vi "Benchmark Delete.vi"() -> ()   [LabVIEW 2017]
uses:
  Source/LookupTable/LookupTable.lvclass/LookupTable.ctl
  3f600695-5b5a-4146-a4af-1e267d96d976.vi
  b6b64ea5-f314-4d4f-8fa7-59ac42c8a07d.vi
  Source/LookupTable/Read Table Reference.vi
  Source/LookupTable/LookupTable.lvclass
panel:
  in  "Table Size":i32=100000
  out "Variant DVR":dbl
  out "Waveform Chart":cluster{dbl, dbl, dbl}(graph)
  out "Variant by value":dbl
  out "Composed Lookup Table":dbl
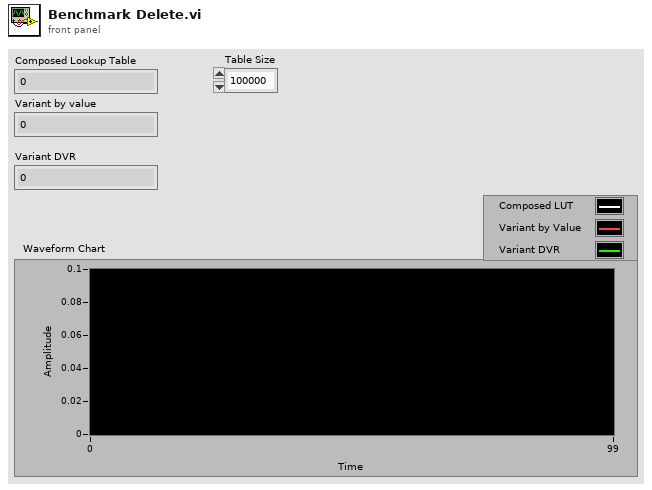
[diagram p1: front panel]
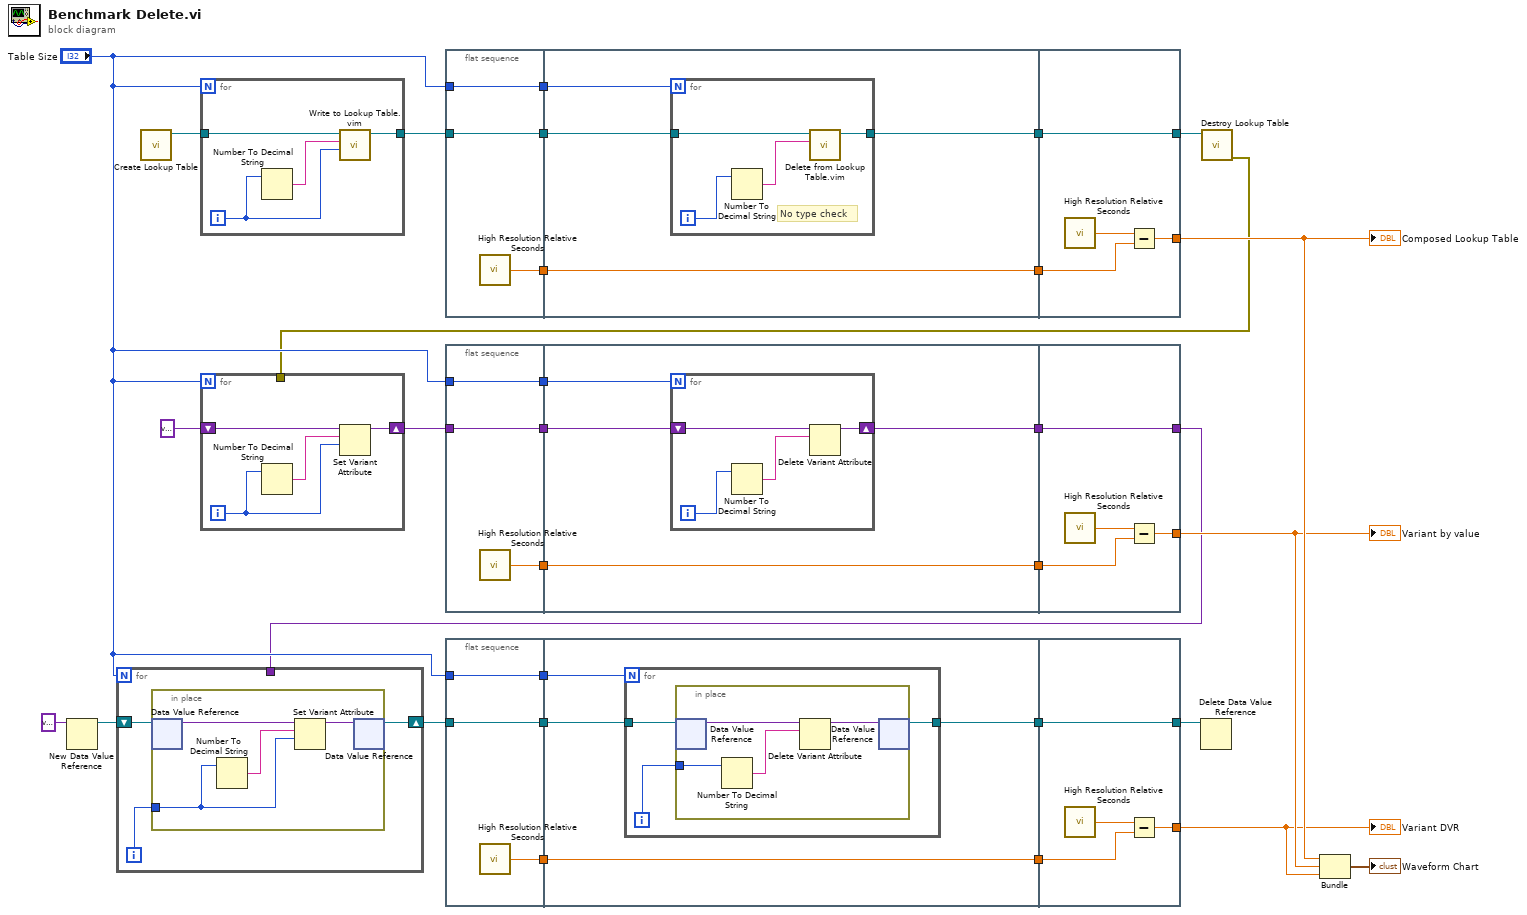
[diagram p0: block diagram]
diagram:
  n1 = New Data Value Reference(data value=variant) -> (data value reference=w12:refnum<data-value>)  [unwired: 1 in, 1 out]
  n2 = for {
    N: "Table Size" -> [_]
    shift-right: [w33] -> w11
    shift-left: w12 -> [w34]
    tunnel: w1 -> [_]
    i -> [w32]
    n3 = in-place {
      in-place-border: w32 -> [w35]
      n4 = in-place-dvr #1(w34) -> (w37:variant)  [unwired: 1 out]
      n5 = Number To Decimal String(number=w35) -> (decimal integer string=w38:string)  [unwired: 1 in]
      n6 = Set Variant Attribute(Variant=w37, name=w38, value=w35) -> (Variant out=w36:variant)  [unwired: 1 in, 2 out]
      n7 = in-place-dvr #1(w36) -> (w33:refnum<data-value>)  [unwired: 1 out]
    }
  }
  n8 = call "Create Lookup Table.vi"() -> ("LookupTable Reference"=w26:refnum<data-value>)  [unwired: 10 in, 1 out]
  n9 = for {
    N: "Table Size" -> [_]
    tunnel: [w40] -> w24
    tunnel: w26 -> [w39]
    i -> [w41]
    n10 = Number To Decimal String(number=w41) -> (decimal integer string=w42:string)  [unwired: 1 in]
    n11 = call "Write to Lookup Table.vim"("Item"=w41, "Item Name"=w42, "LookupTable Reference"=w39) -> ("LookupTable Reference Out"=w40:refnum<data-value>)  [unwired: 6 in, 2 out]
  }
  n12 = flat-sequence {
    tunnel: [w45] -> w31
    tunnel: [w44] -> w25
    tunnel: w24 -> [w44]
    tunnel: [w43] -> w19
    tunnel: "Table Size" -> [w43]
    tunnel: w31 -> [w49]
    tunnel: [w49] -> w30
    tunnel: w25 -> [w48]
    tunnel: [w47] -> w22
    tunnel: w19 -> [w46]
    tunnel: w30 -> [w56]
    tunnel: [w55] -> w9
    tunnel: [w54] -> w23
    tunnel: w22 -> [w54]
    frame #0 {
      n13 = call <vilib>:"High Resolution Relative Seconds.vi"() -> ("relative seconds"=w45:dbl)
    }
    frame #1 {
      n14 = for {
        N: w46 -> [_]
        tunnel: [w51] -> w47
        tunnel: w48 -> [w50]
        i -> [w52]
        # "No type check"
        n15 = Number To Decimal String(number=w52) -> (decimal integer string=w53:string)  [unwired: 1 in]
        n16 = call "Delete from Lookup Table.vim"("Item Name"=w53, "LookupTable Reference"=w50) -> ("LookupTable Reference Out"=w51:refnum<data-value>)  [unwired: 7 in, 2 out]
      }
    }
    frame #2 {
      n17 = call <vilib>:"High Resolution Relative Seconds.vi"() -> ("relative seconds"=w57:dbl)
      n18 = Subtract(x=w57, y=w56) -> (x-y=w55:dbl)
    }
  }
  n19 = flat-sequence {
    tunnel: [w60] -> w29
    tunnel: [w59] -> w21
    tunnel: w20 -> [w59]
    tunnel: "Table Size" -> [w58]
    tunnel: [w58] -> w18
    tunnel: w29 -> [w64]
    tunnel: [w64] -> w28
    tunnel: w21 -> [w63]
    tunnel: w18 -> [w62]
    tunnel: [w61] -> w3
    tunnel: w28 -> [w71]
    tunnel: [w70] -> w8
    tunnel: [w69] -> w1
    tunnel: w3 -> [w69]
    frame #0 {
      n20 = call <vilib>:"High Resolution Relative Seconds.vi"() -> ("relative seconds"=w60:dbl)
    }
    frame #1 {
      n21 = for {
        N: w62 -> [_]
        shift-right: [w68] -> w61
        shift-left: w63 -> [w65]
        i -> [w66]
        n22 = Number To Decimal String(number=w66) -> (decimal integer string=w67:string)  [unwired: 1 in]
        n23 = Delete Variant Attribute(6:w67, 7:w65) -> (3:w68:variant)  [unwired: 1 in, 2 out]
      }
    }
    frame #2 {
      n24 = call <vilib>:"High Resolution Relative Seconds.vi"() -> ("relative seconds"=w72:dbl)
      n25 = Subtract(x=w72, y=w71) -> (x-y=w70:dbl)
    }
  }
  n26 = flat-sequence {
    tunnel: [w75] -> w17
    tunnel: [w74] -> w16
    tunnel: w11 -> [w74]
    tunnel: "Table Size" -> [w73]
    tunnel: [w73] -> w15
    tunnel: w17 -> [w79]
    tunnel: [w79] -> w14
    tunnel: w16 -> [w78]
    tunnel: w15 -> [w76]
    tunnel: [w77] -> w4
    tunnel: w14 -> [w89]
    tunnel: [w88] -> w7
    tunnel: [w87] -> w5
    tunnel: w4 -> [w87]
    frame #0 {
      n27 = call <vilib>:"High Resolution Relative Seconds.vi"() -> ("relative seconds"=w75:dbl)
    }
    frame #1 {
      n28 = for {
        N: w76 -> [_]
        tunnel: [w81] -> w77
        tunnel: w78 -> [w80]
        i -> [w82]
        n29 = in-place {
          in-place-border: w82 -> [w85]
          n30 = in-place-dvr #2(w80) -> (w84:variant)  [unwired: 1 out]
          n31 = Number To Decimal String(number=w85) -> (decimal integer string=w86:string)  [unwired: 1 in]
          n32 = Delete Variant Attribute(6:w86, 7:w84) -> (3:w83:variant)  [unwired: 1 in, 2 out]
          n33 = in-place-dvr #2(w83) -> (w81:refnum<data-value>)  [unwired: 1 out]
        }
      }
    }
    frame #2 {
      n34 = call <vilib>:"High Resolution Relative Seconds.vi"() -> ("relative seconds"=w90:dbl)
      n35 = Subtract(x=w90, y=w89) -> (x-y=w88:dbl)
    }
  }
  n36 = Delete Data Value Reference(data value reference=w5) -> ()  [unwired: 1 in, 2 out]
  n37 = call "Destroy Lookup Table.vi"("LookupTable Reference"=w23) -> ("error out"=w2:errorcluster)  [unwired: 10 in]
  n38 = for {
    N: "Table Size" -> [_]
    shift-right: [w94] -> w20
    shift-left: variant -> [w91]
    tunnel: w2 -> [_]
    i -> [w92]
    n39 = Number To Decimal String(number=w92) -> (decimal integer string=w93:string)  [unwired: 1 in]
    n40 = Set Variant Attribute(Variant=w91, name=w93, value=w92) -> (Variant out=w94:variant)  [unwired: 1 in, 2 out]
  }
  n41 = Bundle(w9, w8, w7) -> (→"Waveform Chart":cluster{dbl, dbl, dbl})  [unwired: 1 in]
  "Composed Lookup Table" <- w9
  "Variant by value" <- w8
  "Variant DVR" <- w7
